vi "HEWH Config Write.vi"(0 "Config File Path":path=path "C:/work/flowconfig.ini", 11 "error in (no error)":errorcluster) -> (15 "error out":errorcluster)   [LabVIEW 2014]
uses:
  Global HEWH.vi
  <vilib>/Utility/config.llb/Write Key (String).vi
  <vilib>/Utility/config.llb/NI_LVConfig.lvlib
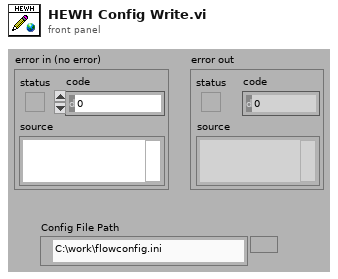
[diagram p1: front panel]
types:
  T1 = typedef "NI_LVConfig.lvlib/Config Data RefNum.ctl" = refnum<k1>
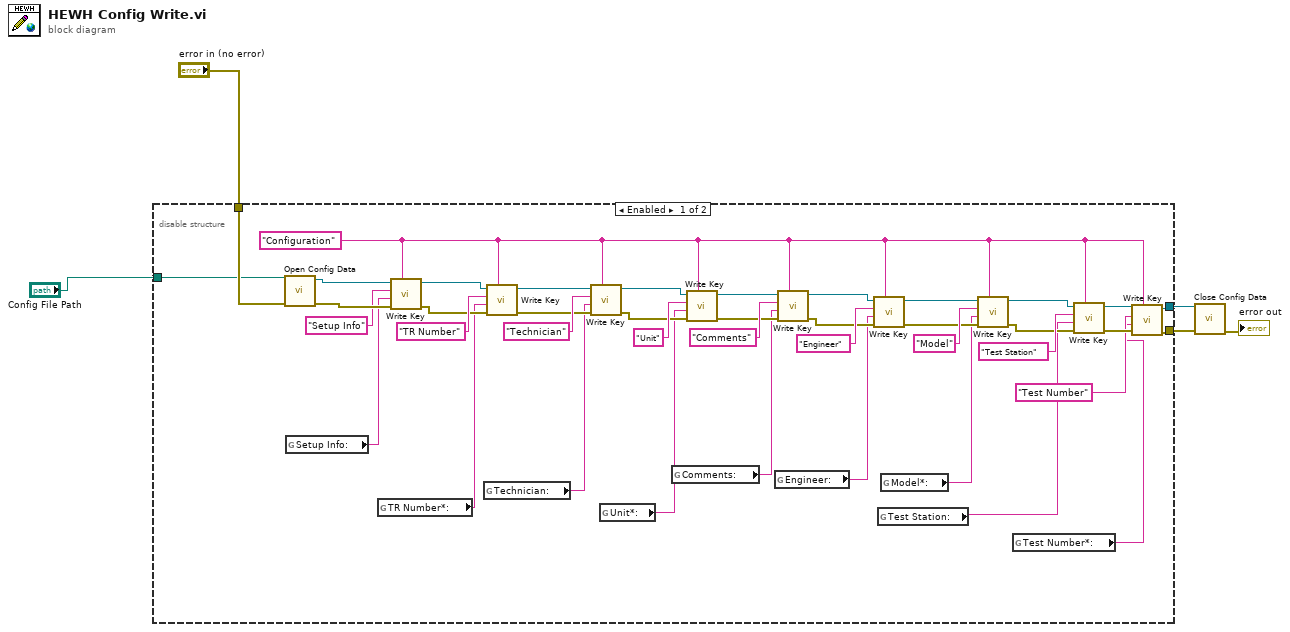
[diagram p0: block diagram]
diagram:
  n1 = disable-structure shown="Enabled" {
    disable-tunnel: "error in (no error)" -> [w45 _]
    disable-tunnel: [w17 _] -> w3
    disable-tunnel: "Config File Path" -> [w21 _]
    disable-tunnel: [w19 _] -> w1
    frame Enabled {
      w16 = "Configuration" ("key")
      n2 = call <vilib>:"Open Config Data.vi"("error in (no error)"=w45, "configuration file path"=w21) -> ("error out"=w44:errorcluster, "refnum"=w46:T1)  [unwired: 7 in, 1 out]
      n3 = global read "Global HEWH.vi" "Setup Info:"() -> (w7:string)
      n4 = global read "Global HEWH.vi" "TR Number*:"() -> (w11:string)
      n5 = call-poly <vilib>:"Write Key.vi"("section"=w16, "error in (no error)"=w44, "value"=w7, "key"="Setup Info", "refnum"=w46) -> ("error out"=w41:errorcluster, "refnum out"=w36:T1)  [unwired: 4 in, 1 out]
      n6 = global read "Global HEWH.vi" "Technician:"() -> (w6:string)
      n7 = call-poly <vilib>:"Write Key.vi"("section"=w16, "error in (no error)"=w41, "value"=w11, "key"="TR Number", "refnum"=w36) -> ("error out"=w37:errorcluster, "refnum out"=w35:T1)  [unwired: 4 in, 1 out]
      n8 = call-poly <vilib>:"Write Key.vi"("section"=w16, "error in (no error)"=w37, "value"=w6, "key"="Technician", "refnum"=w35) -> ("error out"=w38:errorcluster, "refnum out"=w34:T1)  [unwired: 4 in, 1 out]
      n9 = global read "Global HEWH.vi" "Unit*:"() -> (w14:string)
      n10 = global read "Global HEWH.vi" "Comments:"() -> (w8:string)
      n11 = call-poly <vilib>:"Write Key.vi"("section"=w16, "error in (no error)"=w38, "value"=w14, "key"="Unit", "refnum"=w34) -> ("error out"=w22:errorcluster, "refnum out"=w23:T1)  [unwired: 4 in, 1 out]
      n12 = global read "Global HEWH.vi" "Engineer:"() -> (w9:string)
      n13 = call-poly <vilib>:"Write Key.vi"("section"=w16, "error in (no error)"=w22, "value"=w8, "key"="Comments", "refnum"=w23) -> ("error out"=w31:errorcluster, "refnum out"=w26:T1)  [unwired: 4 in, 1 out]
      n14 = call-poly <vilib>:"Write Key.vi"("section"=w16, "error in (no error)"=w31, "value"=w9, "key"="Engineer", "refnum"=w26) -> ("error out"=w27:errorcluster, "refnum out"=w25:T1)  [unwired: 4 in, 1 out]
      n15 = global read "Global HEWH.vi" "Test Station:"() -> (w13:string)
      n16 = global read "Global HEWH.vi" "Model*:"() -> (w10:string)
      n17 = call-poly <vilib>:"Write Key.vi"("section"=w16, "error in (no error)"=w27, "value"=w10, "key"="Model", "refnum"=w25) -> ("error out"=w28:errorcluster, "refnum out"=w24:T1)  [unwired: 4 in, 1 out]
      n18 = global read "Global HEWH.vi" "Test Number*:"() -> (w12:string)
      n19 = call-poly <vilib>:"Write Key.vi"("section"=w16, "error in (no error)"=w28, "value"=w13, "key"="Test Station", "refnum"=w24) -> ("error out"=w18:errorcluster, "refnum out"=w20:T1)  [unwired: 4 in, 1 out]
      n20 = call-poly <vilib>:"Write Key.vi"("section"=w16, "error in (no error)"=w18, "value"=w12, "key"="Test Number", "refnum"=w20) -> ("error out"=w17:errorcluster, "refnum out"=w19:T1)  [unwired: 4 in, 1 out]
    }
    frame Disabled {
    }
  }
  n21 = call <vilib>:"Close Config Data.vi"("error in (no error)"=w3, "refnum"=w1) -> ("error out"=→"error out":errorcluster)  [unwired: 8 in, 1 out]
